vi "test Parameter Add-Find-Remove.vi"(8 "error in":errorcluster, 11 "TestCase in":refnum<class "Scripting.lvclass">) -> (0 "error out":errorcluster, 3 "TestCase out":refnum<class "Scripting.lvclass">)   [LabVIEW 2020, in "Scripting.lvclass"]
uses:
  Scripting.lvclass
  <vilib>/addons/_JKI Toolkits/VI Tester/TestCase.llb/TestCase.lvclass
  Scripting/Ballard/Ballard ARINC 429 Scripting.lvlib
  Shared/Direction.ctl
  <vilib>/NI VeriStand/Custom Device API/Custom Device Item Ref.ctl
  <vilib>/NI VeriStand/Custom Device API/Custom Device API.lvlib
  Shared/SDI.ctl
  <vilib>/NI/NI VeriStand Encoding and Decoding/Encoding.ctl
  <vilib>/NI/NI VeriStand Encoding and Decoding/Encoding and Decoding.lvlib
  Shared/Parameter Definition.ctl
  Shared/Transfer Speed.ctl
  C:/Program Files (x86)/National Instruments/LabVIEW 2020/vi.lib/addons/_JKI Toolkits/VI Tester/TestCase.llb/TestCase.lvclass
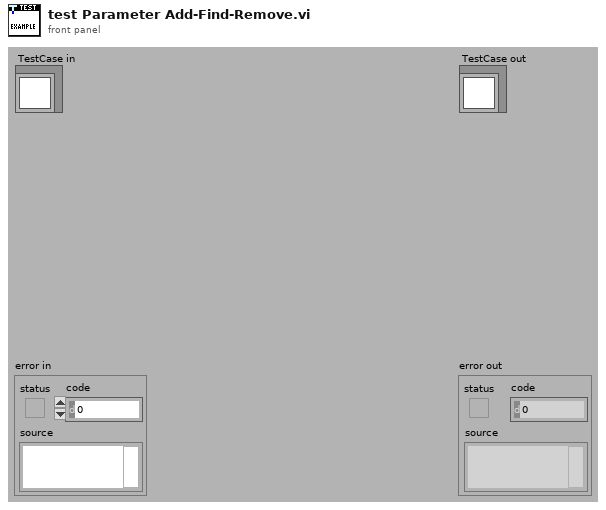
[diagram p1: front panel]
types:
  T1 = typedef "Transfer Speed.ctl" = enum16{"LO (12.5 kb/s)", "HI (100 kb/s)"}
  T2 = cluster{"SDI":bool, "SSM":bool, "Parity":bool, "Timestamp":bool}
  T3 = typedef "Parameter Definition.ctl" = cluster{"start index":i32, "size":i32, "encoding":T4, "signed":bool, "scale multiplier":dbl, "scale offset":dbl}
  T4 = typedef "Encoding and Decoding.lvlib/Encoding.ctl" = enum16{"BNR", "BCD", "Discrete"}
  T5 = typedef "Direction.ctl" = enum16{"Rx", "Tx"}
  T6 = typedef "Custom Device API.lvlib/Custom Device Item Ref.ctl" = u64
  T7 = cluster{"name":string, "unit":string, "default value":dbl}
  T8 = typedef "SDI.ctl" = i32
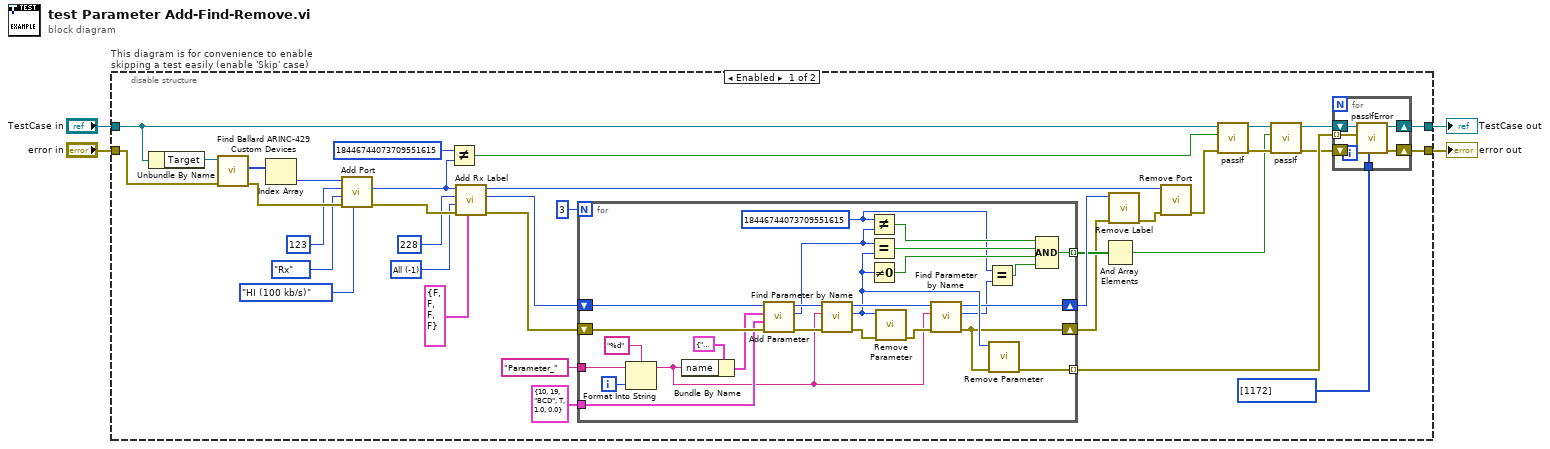
[diagram p0: block diagram]
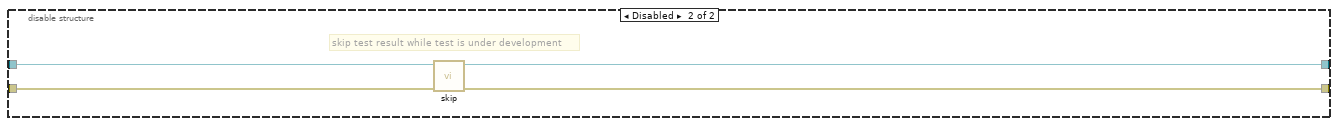
[diagram p2: hidden frame]
diagram:
  n1 = disable-structure "This diagram is for convenience to enable skipping a test easily (enable 'Skip' case)" shown="Enabled" {
    disable-tunnel: "TestCase in" -> [w37 w76]
    disable-tunnel: [w9 w74] -> w1
    disable-tunnel: [w10 w75] -> w3
    disable-tunnel: "error in" -> [w39 w73]
    frame Enabled {
      w32 = T8 -1 items=["All"=-1, "0 (b00)"=0, "1 (b01)"=1, "2 (b10)"=2, "3 (b11)"=3] ("SDI value")
      n2 = Unbundle By Name(w37) -> ("Target"=w40:refnum<k24>)
      n3 = call "Find Ballard ARINC-429 Custom Devices.vi"("error in"=w39, "target in"=w40) -> ("error out"=w30:errorcluster, "Ballard ARINC 429 custom devices"=w38:u64[])  [unwired: 7 in, 1 out]
      n4 = Index Array(array=w38) -> (element=w31:u64)  [unwired: 1 in]
      n5 = call "Add Port.vi"("speed"=Transfer_Speed."HI (100 kb/s)", "error in"=w30, "direction"=Direction."Rx", "port number"=u16 123, "Ballard ARINC 429 custom device in"=w31) -> ("error out"=w36:errorcluster, "port"=w25:T6)  [unwired: 4 in, 1 out]
      n6 = Not Equal?(x=T6 18446744073709551615 ("custom device ref out"), y=w25) -> (x != y?=w26:bool)
      n7 = call "Add Rx Label.vi"("create channels"=T2 {"SDI"=FALSE, "SSM"=FALSE, "Parity"=FALSE, "Timestamp"=FALSE}, "error in"=w36, "SDI value"=w32, "label value"=u32 228, "port in"=w25) -> ("error out"=w19:errorcluster, "label"=w21:T6, "port out"=w35:T6)  [unwired: 4 in]
      n8 = for {
        N: 3 -> [_]
        shift-right: [w52] -> w20
        shift-left: w21 -> [w72]
        shift-right: [w49] -> w15
        shift-left: w19 -> [w66]
        tunnel: T3 {"start index"=10, "size"=19, "encoding"=enum."BCD", "signed"=TRUE, "scale multiplier"=1.0, "scale offset"=0.0} ("parameter definition") -> [w65]
        tunnel: "Parameter_" ("initial string") -> [w62]
        tunnel: [w53] -> w16 mode=indexing
        tunnel: [w48] -> w13 mode=indexing
        i -> [w63]
        w51 = T6 18446744073709551615 ("custom device ref out")
        n9 = Format Into String(format string="%d", initial string=w62, w63) -> (resulting string=w59:string)  [unwired: 1 in, 1 out]
        n10 = Bundle By Name(cluster=T7 {"name"="", "unit"="super units", "default value"=3.0} ("parameter"), "name"=w59) -> (w60:T7)
        n11 = call "Add Parameter.vi"("error in"=w66, "parameter encoding"=w65, "parameter definition"=w60, "label in"=w72) -> ("error out"=w67:errorcluster, "parameter"=w58:T6, "label out"=w71:T6)  [unwired: 5 in]
        n12 = call "Find Parameter by Name.vi"("error in"=w67, "parameter name"=w59, "label in"=w71) -> ("error out"=w68:errorcluster, "parameter ref"=w57:T6, "label out"=w69:T6)  [unwired: 5 in, 1 out]
        n13 = Not Equal?(x=w51, y=w58) -> (x != y?=w55:bool)
        n14 = Equal?(x=w58, y=w57) -> (x = y?=w56:bool)
        n15 = Not Equal To 0?(x=w57) -> (x != 0?=w54:bool)
        n16 = call "Remove Parameter.vi"("error in"=w68, "parameter"=w57) -> ("error out"=w70:errorcluster)  [unwired: 9 in]
        n17 = call "Find Parameter by Name.vi"("error in"=w70, "parameter name"=w59, "label in"=w69) -> ("error out"=w49:errorcluster, "parameter ref"=w47:T6, "label out"=w52:T6)  [unwired: 5 in, 1 out]
        n18 = Equal?(x=w51, y=w47) -> (x = y?=w50:bool)
        n19 = call "Remove Parameter.vi"("error in"=w49, "parameter"=w57) -> ("error out"=w48:errorcluster)  [unwired: 9 in]
        n20 = Compound Arithmetic op=AND(w55, w56, w54, w50) -> (w53:bool)
      }
      n21 = And Array Elements(Boolean array=w16) -> (logical AND=w14:bool)
      n22 = call "Remove Label.vi"("error in"=w15, "label"=w20) -> ("error out"=w24:errorcluster)  [unwired: 9 in]
      n23 = call "Remove Port.vi"("error in"=w24, "port"=w35) -> ("error out"=w7:errorcluster)  [unwired: 9 in]
      n24 = call-dynamic "passIf.vi"("error in (no error)"=w7, "pass"=w26, "TestCase in"=w37) -> ("error out"=w23:errorcluster, "TestCase out"=w34:refnum<class "Scripting.lvclass">)  [unwired: 7 in]
      n25 = call-dynamic "passIf.vi"("error in (no error)"=w23, "pass"=w14, "TestCase in"=w34) -> ("error out"=w11:errorcluster, "TestCase out"=w12:refnum<class "Scripting.lvclass">)  [unwired: 7 in]
      n26 = for {
        tunnel: w13 -> [w46] mode=indexing
        shift-right: [w43] -> w9
        shift-left: w12 -> [w44]
        shift-right: [w42] -> w10
        shift-left: w11 -> [w45]
        tunnel: i32[] [1172] ("passing error codes (default = any error code)") -> [w41]
        n27 = call-dynamic "passIfError.vi"("passing error codes (default = any error code)"=w41, "error in (no error)"=w45, "error"=w46, "TestCase in"=w44) -> ("error out"=w42:errorcluster, "TestCase out"=w43:refnum<class "Scripting.lvclass">)  [unwired: 6 in]
      }
    }
    frame Disabled {
      # "skip test result while test is under development"
      n28 = call <vilib>:"skip.vi"("error in (no error)"=w73, "TestCase in"=w76) -> ("error out"=w75:errorcluster, "TestCase out"=w74:refnum<class "Scripting.lvclass">)  [unwired: 8 in]
    }
  }
  "error out" <- w3
  "TestCase out" <- w1
